vi "D-Type Flip-Flop.vi"(2 "clock":bool, 3 "rest":bool, 4 "Data":bool=TRUE) -> (0 "!Q":bool, 1 "Q":bool=TRUE)   [LabVIEW 2018]
panel:
  # "D-Type\nFlip-Flop"
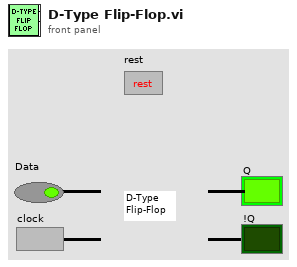
[diagram p1: front panel]
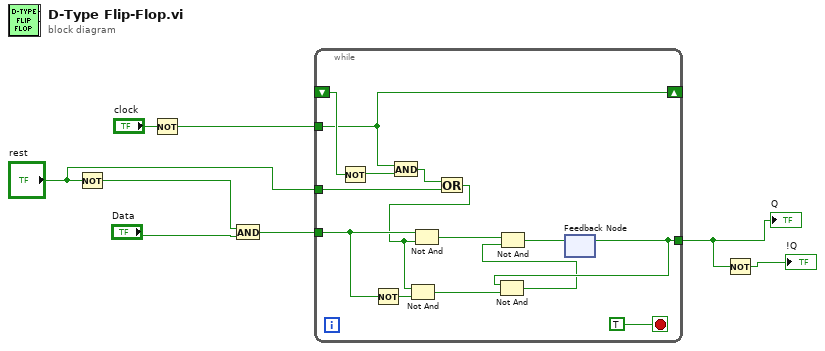
[diagram p0: block diagram]
diagram:
  n1 = Not(x="rest") -> (.not. x?=w2:bool)
  n2 = Not(x="clock") -> (.not. x?=w7:bool)
  n3 = And(x=w2, y="Data") -> (x .and. y?=w4:bool)
  n4 = while {
    shift-right: [w19] -> _
    shift-left: _ -> [w21]
    tunnel: w7 -> [w19]
    tunnel: w4 -> [w17]
    tunnel: [w13] -> w5
    tunnel: "rest" -> [w10]
    stop <- TRUE stop-if-true
    n5 = Not(x=w21) -> (.not. x?=w20:bool)
    n6 = Not(x=w17) -> (.not. x?=w18:bool)
    n7 = And(x=w19, y=w20) -> (x .and. y?=w11:bool)
    n8 = Or(x=w11, y=w10) -> (x .or. y?=w9:bool)
    n9 = Not And(1:w18, 2:w9) -> (0:w15:bool)
    n10 = Not And(1:w9, 2:w17) -> (0:w16:bool)
    n11 = feedback #1() -> (w13:bool)  [unwired: 1 in]
    n12 = Not And(1:w15, 2:w13) -> (0:w12:bool)
    n13 = Not And(1:w12, 2:w16) -> (0:w14:bool)
    n14 = feedback-in #1(w14) -> ()
  }
  "Q" <- w5
  n15 = Not(x=w5) -> (.not. x?=→"!Q":bool)
